vi "CleanUp.vi"(8 "error in (no error)":errorcluster, 11 "Color in":refnum<class "Color.lvclass">) -> (0 "error out":errorcluster, 3 "Color out":refnum<class "Color.lvclass">)   [LabVIEW 2020]
uses:
  Color.lvclass
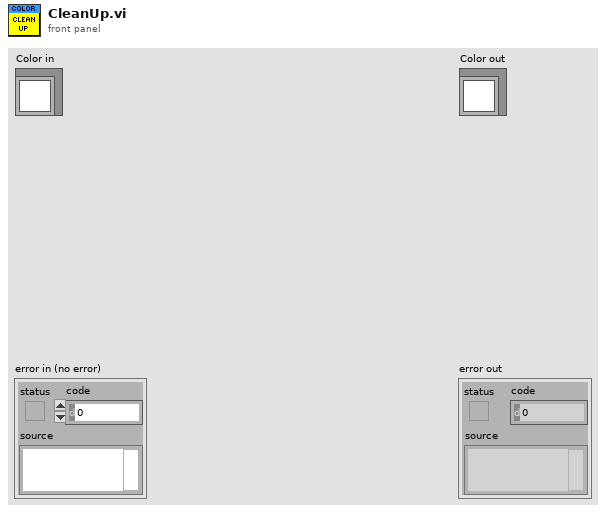
[diagram p1: front panel]
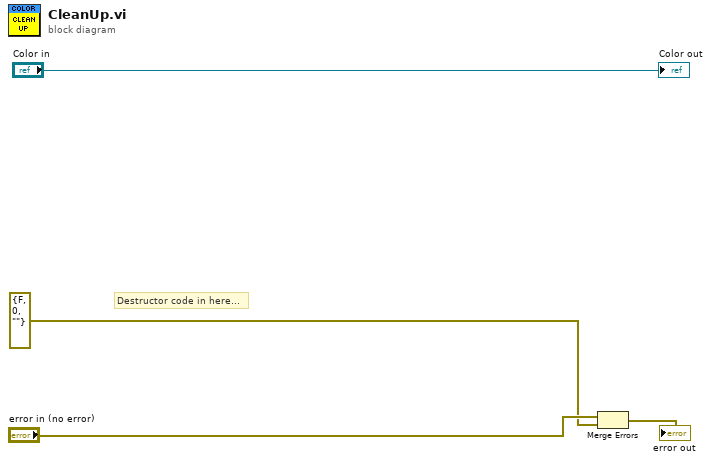
[diagram p0: block diagram]
diagram:
  # "Destructor code in here..."
  n1 = Merge Errors("error in (no error)", errorcluster {"status"=FALSE, "code"=0, "source"=""} ("error in (no error)")) -> (→"error out":errorcluster)
  "Color out" <- "Color in"
